vi "Configure Signaling Additional Spectrum Emission.vi"(8 "error in (no error)":errorcluster, 9 "Additional Spectrum Emission (1)":i32=1, 10 "Cell Name (\"Cell Name\")":string="Cell Name", 11 "VISA resource name":refnum<visa-resource-name>) -> (0 "error out":errorcluster, 3 "VISA resource name out":refnum<visa-resource-name>)   [LabVIEW 2020, in "Rohde&Schwarz CMWXP NR FR1 Measurement.lvlib"]
doc: "Sets the parameter 'AdditionalSpectrumEmission', signaled to the UE if the value is not OFF.\n\nAttribute:\nRSCMWXPNRFR1M_ATTR_SIGNALING_ADDITIONAL_SPECTRUM_EMISSION\n\nRemote-control command:\n[CONFigure:]SIGNaling:NRADio:CELL:RFSettings:ASEMission"
uses:
  <instrlib>/Rohde&Schwarz CMWXP NR FR1 Measurement/Rohde&Schwarz CMWXP NR FR1 Measurement.lvlib
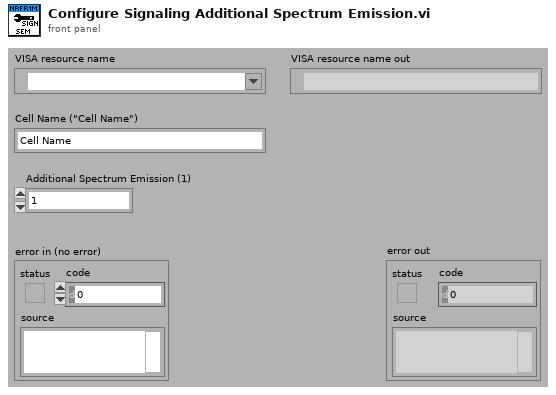
[diagram p1: front panel]
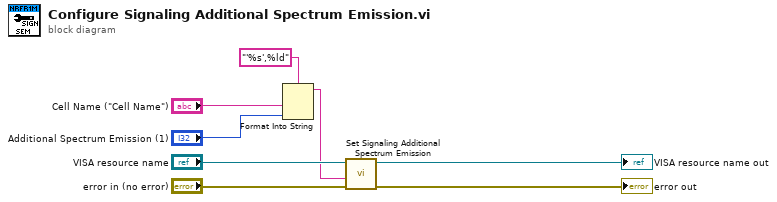
[diagram p0: block diagram]
diagram:
  n1 = Format Into String(format string="'%s',%ld", "Cell Name (\"Cell Name\")", "Additional Spectrum Emission (1)") -> (resulting string=w1:string)  [unwired: 2 in, 1 out]
  n2 = call "Set Signaling Additional Spectrum Emission"("error in (no error)"="error in (no error)", "Signaling Additional Spectrum Emission ()"=w1, "instrument handle"="VISA resource name") -> ("error out"=→"error out":errorcluster, "instrument handle out"=→"VISA resource name out":refnum<visa-resource-name>)  [unwired: 7 in]
